vi "Get Array Size.vi"(2 "error in (no error)":errorcluster, 3 "JSON Array in":refnum<class "JSON Helper.lvclass">) -> (0 "error out":errorcluster, 1 "size(s)":i32)   [LabVIEW 2016, in "JSON Helper.lvclass"]
doc: "Returns the number of elements in a JSON Array"
uses:
  JSON Helper/JSON Helper.lvclass
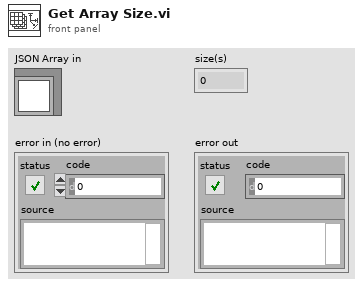
[diagram p1: front panel]
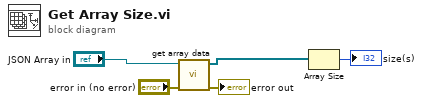
[diagram p0: block diagram]
diagram:
  n1 = call "get array data.vi"("error in (no error)"="error in (no error)", "JSON Helper in"="JSON Array in") -> ("error out"=→"error out":errorcluster, "JSON Array out"=w3:refnum<class "JSON Helper.lvclass">[])  [unwired: 8 in]
  n2 = Array Size(array=w3) -> (size(s)=→"size(s)":i32)
